vi "IMAQController.SetNewController.vi"(1 "Array":refnum<notifier>[](array[refnum]), 5 "error in":errorcluster) -> (15 "Controller Array":string[](array[string]), 17 "new list?":bool, 19 "error out":errorcluster)   [LabVIEW 2014]
uses:
  CSlibraries-extern/DimLVEvent/LVDimInterface/LVDimInterface.lvlib
  CSCore/CSSystem/CoreLib/CoreLib.lvlib
  CSCore/CSSystem/CSSystemLib/CSSystemLib.lvlib
panel:
  out "Array 4":bool[][](array[boolean])
  out "Array 3":bool[](array[boolean])
  out "Array 2":string[][](array[string])
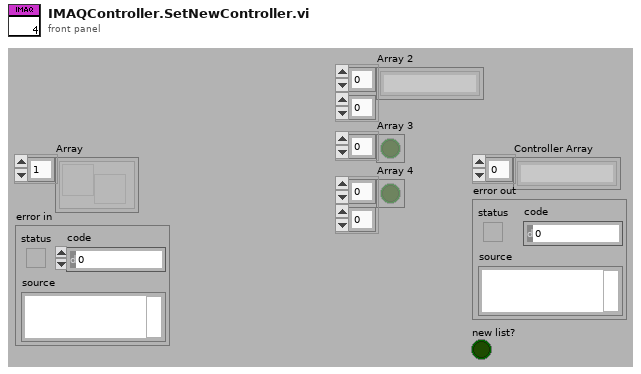
[diagram p1: front panel]
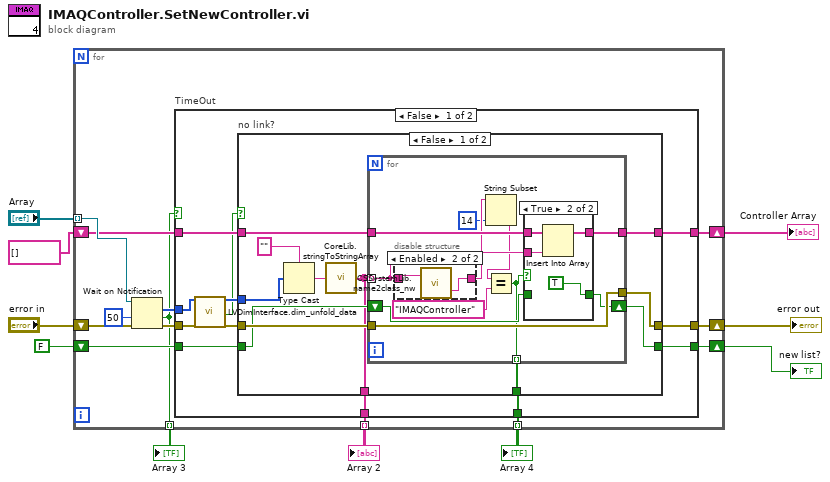
[diagram p0: block diagram]
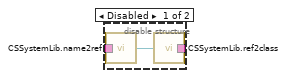
[diagram p2: hidden frame]
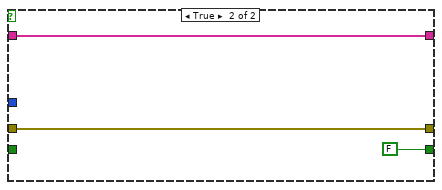
[diagram p4: hidden frame]
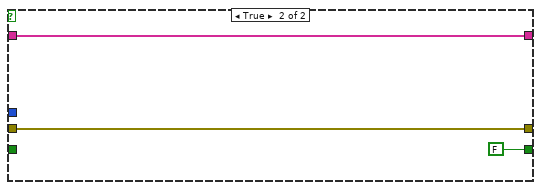
[diagram p5: hidden frame]
diagram:
  n1 = for {
    tunnel: "Array" -> [w23] mode=indexing
    shift-right: [w19] -> w7
    shift-left: string[] [] -> [w20]
    shift-right: [w17] -> w5
    shift-left: "error in" -> [w18]
    shift-right: [w15] -> w6
    shift-left: FALSE -> [w16]
    tunnel: [w13] -> w3 mode=indexing
    tunnel: [w12] -> w2 mode=indexing
    tunnel: [w11] -> w1 mode=indexing
    n2 = Wait on Notification(notifier=w23, timeout in ms (-1)=50, error in (no error)=w18) -> (notification=w22:i8[], timed out?=w12:bool, error out=w21:errorcluster)  [unwired: 1 in, 1 out]
    n3 = case "TimeOut" shown="False" w12 {
      tunnel: w22 -> [w35 _]
      tunnel: w21 -> [w33 w73]
      tunnel: w20 -> [w32 w74]
      tunnel: [w31 w74] -> w19
      tunnel: [w29 w73] -> w17
      tunnel: w16 -> [w28 _]
      tunnel: [w27 FALSE] -> w15
      tunnel: [w25 _] -> w13
      tunnel: [w24 _] -> w11
      frame False {
        n4 = call "LVDimInterface.dim_unfold_data.vi"("rawData"=w35, "error in (no error)"=w33) -> ("data"=w34:i8[], "no link"=w26:bool, "error out"=w30:errorcluster)  [unwired: 14 in, 1 out]
        n5 = case "no link?" shown="False" w26 {
          tunnel: w34 -> [w46 _]
          tunnel: w32 -> [w43 w69]
          tunnel: [w42 w69] -> w31
          tunnel: w30 -> [w41 w70]
          tunnel: [w40 w70] -> w29
          tunnel: w28 -> [w39 _]
          tunnel: [w38 FALSE] -> w27
          tunnel: [w37 _] -> w25
          tunnel: [w36 _] -> w24
          frame False {
            n6 = Type Cast(type="", x=w46) -> (*(type *) &x=w44:string)
            n7 = call "CoreLib.stringToStringArray.vi"("String"=w44) -> ("Array"=w37:string[])
            n8 = for {
              tunnel: w37 -> [w54] mode=indexing
              tunnel: w43 -> [w56]
              tunnel: [w55] -> w42
              tunnel: w41 -> [w53]
              tunnel: [w53] -> w40
              shift-right: [w51] -> w38
              shift-left: w39 -> [w52]
              tunnel: [w50] -> w36 mode=indexing
              n9 = disable-structure shown="Enabled" {
                disable-tunnel: [w59 w62] -> w49
                disable-tunnel: w54 -> [w58 w61]
                frame Disabled {
                  n10 = call "CSSystemLib.name2ref.vi"("name"=w58) -> ("obj refnum"=w60:refnum<vi>)
                  n11 = call "CSSystemLib.ref2class.vi"("obj refnum"=w60) -> ("class"=w59:string)
                }
                frame Enabled {
                  n12 = call "CSSystemLib.name2class_nw.vi"("name"=w61) -> ("classID"=w62:string)  [unwired: 16 in, 2 out]
                }
              }
              n13 = String Subset(string=w49, length (rest)=14 ("length (rest)")) -> (substring=w48:string)  [unwired: 1 in]
              n14 = Equal?(x=w48, y="IMAQController") -> (x = y?=w50:bool)
              n15 = case shown="True" w50 {
                tunnel: w56 -> [w64 w68]
                tunnel: [w64 w67] -> w55
                tunnel: w54 -> [_ w66]
                tunnel: w52 -> [w63 _]
                tunnel: [w63 TRUE] -> w51
                frame False {
                }
                frame True {
                  n16 = Insert Into Array(array=w68, new element=w66) -> (w67:string[])  [unwired: 1 in]
                }
              }
            }
          }
          frame True {
          }
        }
      }
      frame True {
      }
    }
  }
  "Controller Array" <- w7
  "new list?" <- w6
  "error out" <- w5
  "Array 2" <- w3
  "Array 3" <- w2
  "Array 4" <- w1
